vi "radial-profile-centerR-range-complex.vi"(4 "num":i32=2, 6 "R-step":sgl=1.0, 8 "error in (no error)":errorcluster caption="错误输入（无错误）", 9 "R-min":sgl, 10 "R-max":sgl, 11 "Complex Image Src":T1) -> (0 "error out":errorcluster caption="错误输出", 1 "profile-r":dbl[](array[numeric]), 2 "ArrayR":sgl[](array[numeric]))   [LabVIEW 2013]
uses:
  <vilib>/vision/Image Controls.llb/IMAQ Image.ctl
  <vilib>/vision/NI_Vision_Development_Module.lvlib
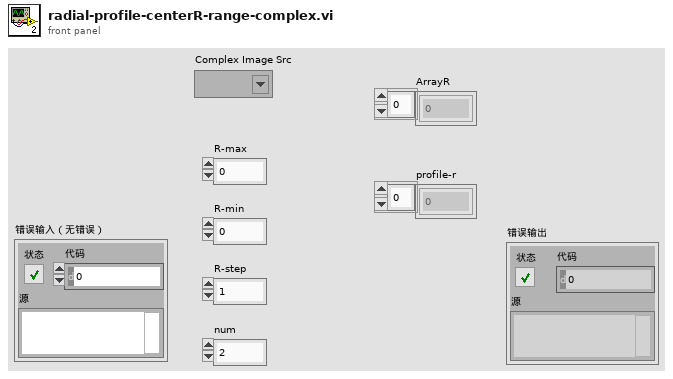
[diagram p1: front panel]
types:
  T1 = typedef "IMAQ Image.ctl" = refnum<image>
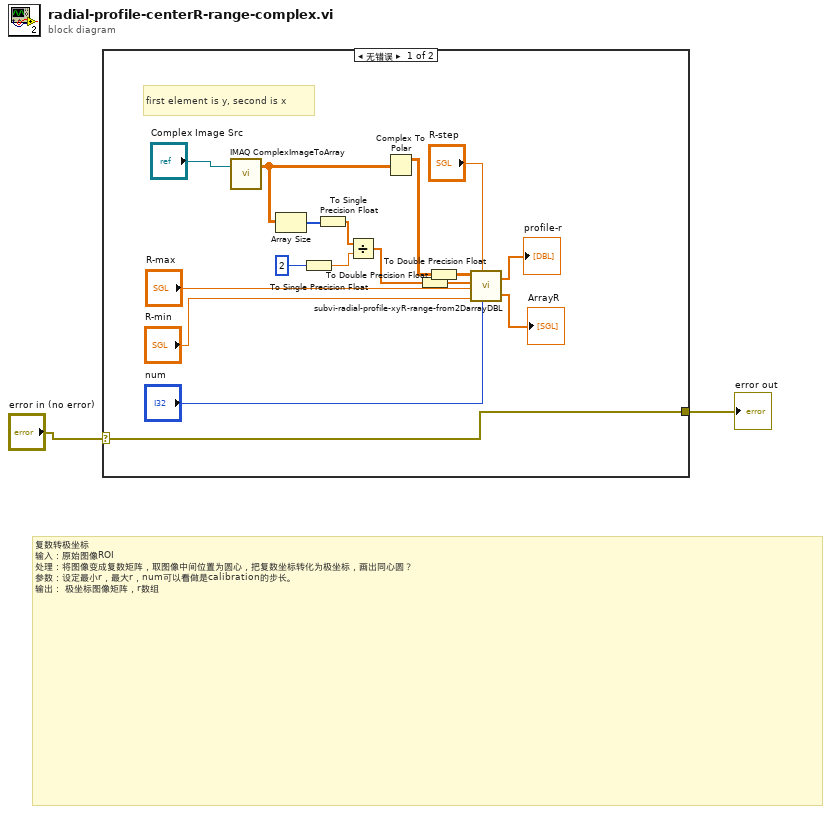
[diagram p0: block diagram]
diagram:
  # "复数转极坐标\n输入：原始图像ROI\n处理：将图像变成复数矩阵，取图像中间位置为圆心，把复数坐标转化为极坐标，画出同心圆？\n参数：设定最小r，最大r，num可以看做是calibration的步长。\n输出： 极坐标图像矩阵，r数组"
  n1 = case shown="无错误" "error in (no error)" {
    selector: "error in (no error)" -> [w3 w20]
    tunnel: [w3 w20] -> w1
    frame No Error {
      # "first element is y, second is x"
      n2 = call "IMAQ ComplexImageToArray"("Image"="Complex Image Src") -> ("Image Pixels (Complex)"=w17:csg[][])  [unwired: 2 in, 3 out]
      n3 = Array Size(array=w17) -> (size(s)=w16:i32[])
      n4 = To Single Precision Float(number=2) -> (single precision float=w6:sgl)
      n5 = To Single Precision Float(number=w16) -> (single precision float=w7:sgl[])
      n6 = Divide(x=w7, y=w6) -> (x/y=w13:sgl[])
      n7 = Complex To Polar(r * e^(i*theta)=w17) -> (r=w14:sgl[][])  [unwired: 1 out]
      n8 = To Double Precision Float(number=w13) -> (double precision float=w4:dbl[])
      n9 = To Double Precision Float(number=w14) -> (double precision float=w5:dbl[][])
      n10 = call "subvi-radial-profile-xyR-range-from2DarrayDBL.vi"("num"="num", "R-step"="R-step", "R-min"="R-min", "R-max"="R-max", "y/x"=w4, "2D array"=w5) -> ("ArrayR"=→"ArrayR":sgl[], "profile"=→"profile-r":dbl[])
    }
    frame Error {
    }
  }
  "error out" <- w1
